vi "obtainSALLVFunctionReferences.vi"(8 "error in (no error)":errorcluster, 11 "enterControl in":refnum<class "enterControl.lvclass">) -> (0 "error out":errorcluster, 3 "enterControl out":refnum<class "enterControl.lvclass">)   [LabVIEW 2016, in "SALLV_AtDome_Messaging.lvlib" / "enterControl.lvclass"]
uses:
  enterControl.lvclass
  home/andres/ts_AtDome/SALTopic/SALTopic/SALTopic.lvclass
  enterControl.lvclass/enterControl.ctl
  SALTopic/SALCommand/SALCommand.lvclass
  SALTopic/SALTopic/SALTopic.lvclass
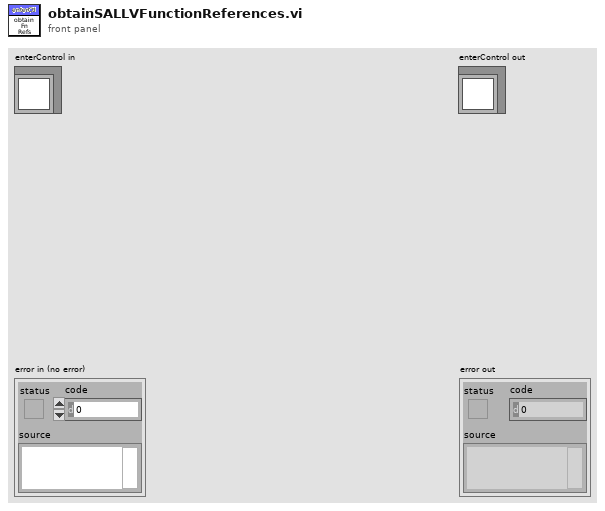
[diagram p1: front panel]
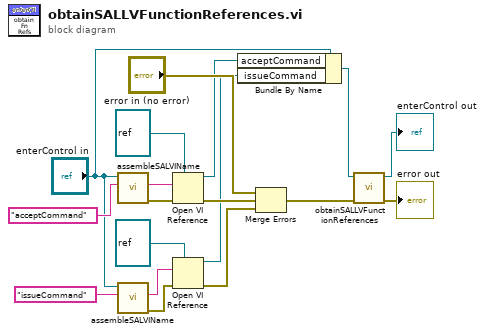
[diagram p0: block diagram]
diagram:
  n1 = call "assembleSALVIName.vi"("topicKey"="acceptCommand" ("commandKey"), "SALTopic in"="enterControl in") -> ("error out"=w14:errorcluster, "viPath"=w15:string)  [unwired: 7 in, 1 out]
  n2 = call "assembleSALVIName.vi"("topicKey"="issueCommand" ("commandKey"), "SALTopic in"="enterControl in") -> ("error out"=w11:errorcluster, "viPath"=w10:string)  [unwired: 7 in, 1 out]
  n3 = Open VI Reference(type specifier VI Refnum (for type only)=refnum<vi> refnum ("reference"), vi path=w15, error in (no error)=w14) -> (vi reference=w4:refnum<vi>, error out=w7:errorcluster)  [unwired: 3 in]
  n4 = Open VI Reference(type specifier VI Refnum (for type only)=refnum<vi> refnum ("reference"), vi path=w10, error in (no error)=w11) -> (vi reference=w3:refnum<vi>, error out=w6:errorcluster)  [unwired: 3 in]
  n5 = Bundle By Name(cluster="enterControl in", "acceptCommand"=w4, "issueCommand"=w3) -> (w2:refnum<class "enterControl.lvclass">)
  n6 = Merge Errors("error in (no error)", w7, w6) -> (w1:errorcluster)
  n7 = call-parent "obtainSALLVFunctionReferences.vi"("error in (no error)"=w1, "SALCommand in"=w2) -> ("error out"=→"error out":errorcluster, "SALCommand out"=→"enterControl out":refnum<class "enterControl.lvclass">)  [unwired: 8 in]
